vi "Motors Interface.vi"() -> ()   [LabVIEW 2011]
uses:
  Controls/Drive Status.ctl
  <vilib>/LabVIEW Targets/FPGA/cRIO/cRIO-9505/controls.llb/_nicrio_cRIO-9505_DriveStatus.ctl
  <vilib>/Platform/TimedLoop/XDataNode/timing_clust.ctl
  <vilib>/Platform/TimedLoop/XDataNode/nitl_modes.ctl
  <vilib>/Platform/TimedLoop/XDataNode/wakeup.ctl
  Controls/Motor Names.ctl
  Controls/Motor Module.ctl
  Controls/Encoder Module.ctl
  <vilib>/Platform/TimedLoop/XDataNode/XDataNode.xnode
  <vilib>/Platform/TimedLoop/XDataNode/XDNodeRunTimeDep.lvlib
panel:
  in  "tikcs before":i16=10
  out "Current Index 3":i16
  out "Current Index 2":i16
  out "Current Index 1":i16
  out "Current Middle 3":i16
  out "Current Middle 2":i16
  out "Current Middle 1":i16
  out "Current Redundant":i16
  out "Current Thumb 3":i16
  out "Current Thumb 2":i16
  out "Current Thumb 1":i16
  out "Motors Status":T1[](array[typedef])=[{"Status"=enum."Enabled", "Vsup Present"=FALSE, "Drive Fault"=FALSE, "Temp Fault"=FALSE}, {"Status"=enum."Enabled", "Vsup Present"=FALSE, "Drive Fault"=FALSE, "Temp Fault"=FALSE}, {"Status"=enum."Enabled", "Vsup Present"=FALSE, "Drive Fault"=FALSE, "Temp Fault"=FALSE}, {"Status"=enum."Enabled", "Vsup Present"=FALSE, "Drive Fault"=FALSE, "Temp Fault"=FALSE}, {"Status"=enum."Enabled", "Vsup Present"=FALSE, "Drive Fault"=FALSE, "Temp Fault"=FALSE}, {"Status"=enum."Enabled", "Vsup Present"=FALSE, "Drive Fault"=FALSE, "Temp Fault"=FALSE}, {"Status"=enum."Enabled", "Vsup Present"=FALSE, "Drive Fault"=FALSE, "Temp Fault"=FALSE}, {"Status"=enum."Enabled", "Vsup Present"=FALSE, "Drive Fault"=FALSE, "Temp Fault"=FALSE}, {"Status"=enum."Enabled", "Vsup Present"=FALSE, "Drive Fault"=FALSE, "Temp Fault"=FALSE}, {"Status"=enum."Enabled", "Vsup Present"=FALSE, "Drive Fault"=FALSE, "Temp Fault"=FALSE}]
  out "Position Middle 3":i32
  in  "Current Limit Middle 3":i16 caption="Setpoint"
  in  "Current Setpoint Middle 3":i16
  out "Position Middle 2":i32
  in  "Current Limit Middle 2":i16 caption="Setpoint"
  in  "Current Setpoint Middle 2":i16
  out "Position Middle 1":i32
  in  "Current Limit Middle 1":i16 caption="Setpoint"
  in  "Current Setpoint Middle 1":i16
  out "Position Redundant":i32
  in  "Current Limit Redundant":i16 caption="Setpoint"
  in  "Current Setpoint Redundant":i16
  out "Position Thumb 3":i32
  in  "Current Limit Thumb 3":i16 caption="Setpoint"
  in  "Current Setpoint Thumb 3":i16
  out "Position Thumb 2":i32
  in  "Current Limit Thumb 2":i16 caption="Setpoint"
  in  "Current Setpoint Thumb 2":i16
  out "Position Thumb 1":i32
  in  "Current Limit Thumb 1":i16 caption="Setpoint"
  in  "Current Setpoint Thumb 1":i16
  out "Position Index 3":i32
  in  "Current Limit Index 3":i16 caption="Setpoint"
  in  "Current Setpoint Index 3":i16
  out "Position Index 2":i32
  in  "Current Limit Index 2":i16 caption="Setpoint"
  in  "Current Setpoint Index 2":i16
  out "Position Index 1":i32
  in  "Current Limit Index 1":i16 caption="Setpoint"
  in  "Rate (usec)":u32=50
  in  "Motors Gains":T3={"Proportional Gain"=20, "Integral Gain"=10, "Derivative Gain"=0}
  in  "Current Setpoint Index 1":i16
  out "All Enabled":bool
  in  "Disable\nMotors":bool
  in  "Enable\nMotors":bool
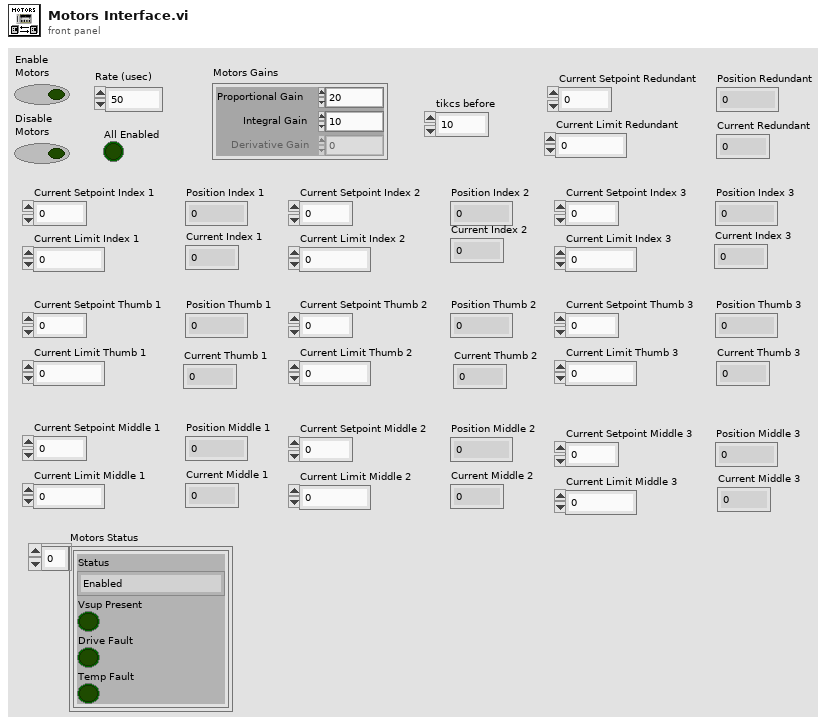
[diagram p1: front panel]
types:
  T1 = typedef "Drive Status.ctl" = cluster{"Status":T2, "Vsup Present":bool, "Drive Fault":bool, "Temp Fault":bool}
  T2 = typedef "_nicrio_cRIO-9505_DriveStatus.ctl" = enum8{"Enabled", "Disabled", "Disabled by Drive Fault", "Disabled by Temp. Fault", "Disabled by E-Stop", "Unknown"}
  T3 = cluster{"Proportional Gain":i16, "Integral Gain":i16, "Derivative Gain":i16}
  T4 = typedef "Motor Names.ctl" = enum16{"Thumb1", "Thumb2", "Thumb3", "Middle1", "Middle2", "Middle3", "Redundant", "Index1", "Index2", "Index3"}
  T5 = typedef "XDNodeRunTimeDep.lvlib/timing_clust.ctl" = cluster{"Expected End [f-1]":u64, "Actual End [f-1]":u64, "Finished Late? [f-1]":bool, "Expected End [i-1]":u64, "Actual End [i-1]":u64, "Finished Late? [i-1]":bool, "Expected Start [i]":u64, "Actual Start [i]":u64, "Expected Start [f]":u64, "Actual Start [f]":u64, "Source Name":string, "Structure Name":string, "Period":i64, "Deadline":i64, "Offset":i64, "Start":i64, "Priority":i32, "Timeout":i32, "Mode":T6, "Wakeup Reason":T7, "Error":errorcluster, "Source Type":string, "Secondary Source Type":string, "Global End Time":u64, "Global Start Time":u64, "Frame Duration":u64, "Iteration Duration":u64, "Assigned CPU":i32, "I/O Scan Engine Mode":u32}
  T6 = typedef "XDNodeRunTimeDep.lvlib/nitl_modes.ctl" = enum32{"No Change", "Process missed periods, maintain original phase", "Discard missed periods, maintain original phase", "Process missed periods, ignore original phase", "Discard missed periods, ignore original phase"}
  T7 = typedef "XDNodeRunTimeDep.lvlib/wakeup.ctl" = enum32{"Normal", "Aborted", "Asynchronous wakeup", "Timing source error", "Timed loop error", "Timeout"}
  T8 = typedef "Encoder Module.ctl" = cluster{"Encoder Phase A":refnum<k21>, "Encoder Phase B":refnum<k21>, "Encoder Index":refnum<k21>}
  T9 = typedef "Motor Module.ctl" = cluster{"Motor":refnum<k21>, "Drive Direction":refnum<k21>}
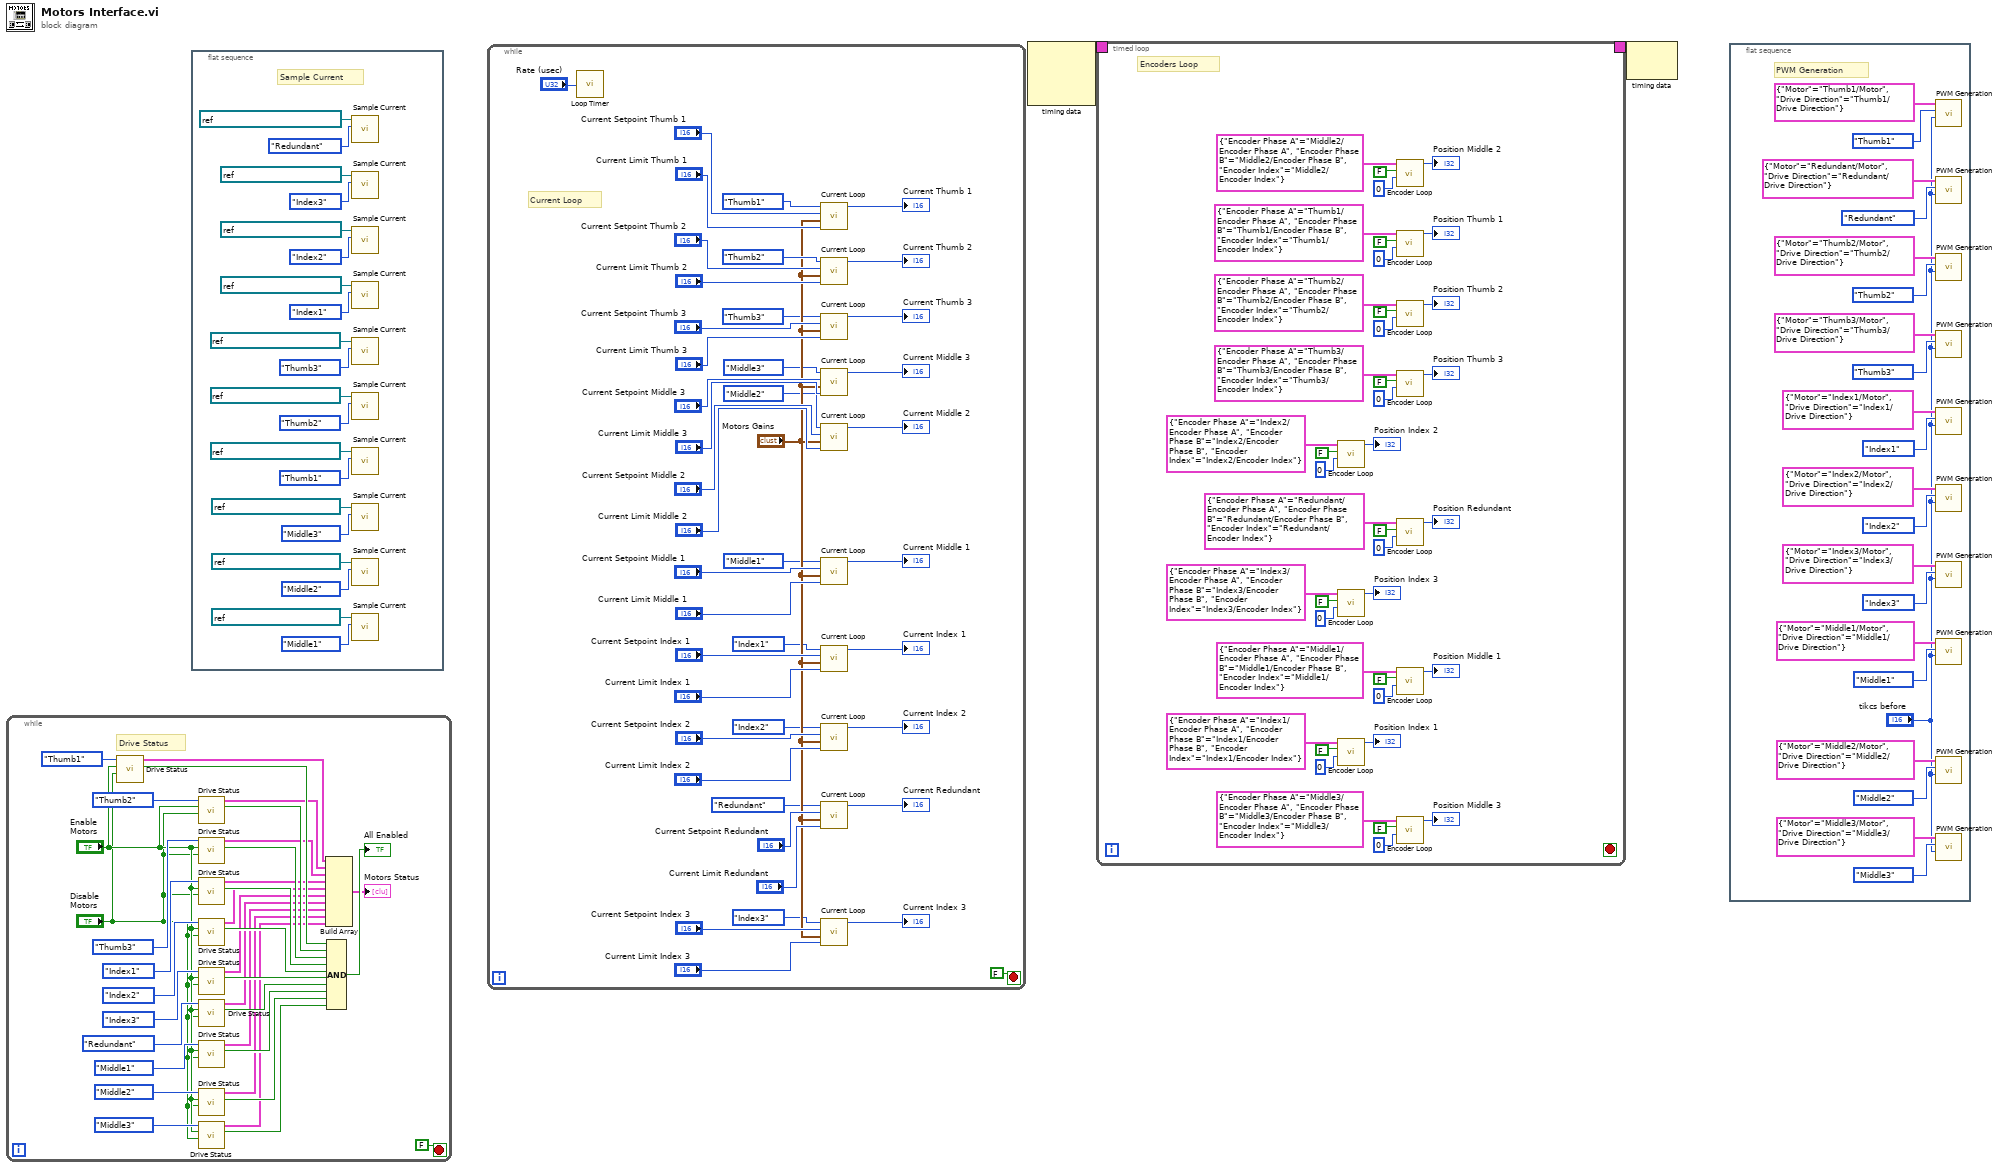
[diagram p0: block diagram]
diagram:
  n1 = while {
    stop <- FALSE stop-if-true
    # "Drive Status"
    n2 = call "Drive Status.vi"("Disable\nDrive"="Disable\nMotors", "Enable\nDrive"="Enable\nMotors", "Motor"=Motor_Names."Thumb1") -> ("Enabled?"=w24:bool, "Drive Status"=w14:T1)  [unwired: 7 in]
    n3 = call "Drive Status.vi"("Disable\nDrive"="Disable\nMotors", "Enable\nDrive"="Enable\nMotors", "Motor"=Motor_Names."Thumb2") -> ("Enabled?"=w23:bool, "Drive Status"=w13:T1)  [unwired: 7 in]
    n4 = call "Drive Status.vi"("Disable\nDrive"="Disable\nMotors", "Enable\nDrive"="Enable\nMotors", "Motor"=Motor_Names."Thumb3") -> ("Enabled?"=w22:bool, "Drive Status"=w12:T1)  [unwired: 7 in]
    n5 = call "Drive Status.vi"("Disable\nDrive"="Disable\nMotors", "Enable\nDrive"="Enable\nMotors", "Motor"=Motor_Names."Index1") -> ("Enabled?"=w21:bool, "Drive Status"=w11:T1)  [unwired: 7 in]
    n6 = call "Drive Status.vi"("Disable\nDrive"="Disable\nMotors", "Enable\nDrive"="Enable\nMotors", "Motor"=Motor_Names."Index2") -> ("Enabled?"=w20:bool, "Drive Status"=w10:T1)  [unwired: 7 in]
    n7 = call "Drive Status.vi"("Disable\nDrive"="Disable\nMotors", "Enable\nDrive"="Enable\nMotors", "Motor"=Motor_Names."Index3") -> ("Enabled?"=w19:bool, "Drive Status"=w9:T1)  [unwired: 7 in]
    n8 = call "Drive Status.vi"("Disable\nDrive"="Disable\nMotors", "Enable\nDrive"="Enable\nMotors", "Motor"=Motor_Names."Redundant") -> ("Enabled?"=w18:bool, "Drive Status"=w8:T1)  [unwired: 7 in]
    n9 = call "Drive Status.vi"("Disable\nDrive"="Disable\nMotors", "Enable\nDrive"="Enable\nMotors", "Motor"=Motor_Names."Middle1") -> ("Enabled?"=w17:bool, "Drive Status"=w7:T1)  [unwired: 7 in]
    n10 = call "Drive Status.vi"("Disable\nDrive"="Disable\nMotors", "Enable\nDrive"="Enable\nMotors", "Motor"=Motor_Names."Middle2") -> ("Enabled?"=w16:bool, "Drive Status"=w6:T1)  [unwired: 7 in]
    n11 = call "Drive Status.vi"("Disable\nDrive"="Disable\nMotors", "Enable\nDrive"="Enable\nMotors", "Motor"=Motor_Names."Middle3") -> ("Enabled?"=w15:bool, "Drive Status"=w5:T1)  [unwired: 7 in]
    n12 = Build Array(w14, w13, w12, w11, w10, w9, w8, w7, w6, w5) -> (→"Motors Status":T1[])
    n13 = Compound Arithmetic op=AND(w24, w23, w22, w21, w20, w19, w18, w17, w16, w15) -> (→"All Enabled":bool)
  }
  n14 = flat-sequence {
    frame #0 {
      # "Sample Current"
      n15 = call "Sample Current.vi"("Motor Index"=Motor_Names."Redundant" ("Motor Names"), "Current Sense I/O"=refnum<k21> "Redundant/Current Sense") -> ()  [unwired: 10 in]
      n16 = call "Sample Current.vi"("Motor Index"=Motor_Names."Index3" ("Motor Names"), "Current Sense I/O"=refnum<k21> "Index3/Current Sense") -> ()  [unwired: 10 in]
      n17 = call "Sample Current.vi"("Motor Index"=Motor_Names."Index2" ("Motor Names"), "Current Sense I/O"=refnum<k21> "Index2/Current Sense") -> ()  [unwired: 10 in]
      n18 = call "Sample Current.vi"("Motor Index"=Motor_Names."Index1" ("Motor Names"), "Current Sense I/O"=refnum<k21> "Index1/Current Sense") -> ()  [unwired: 10 in]
      n19 = call "Sample Current.vi"("Motor Index"=Motor_Names."Thumb3" ("Motor Names"), "Current Sense I/O"=refnum<k21> "Thumb3/Current Sense") -> ()  [unwired: 10 in]
      n20 = call "Sample Current.vi"("Motor Index"=Motor_Names."Thumb2" ("Motor Names"), "Current Sense I/O"=refnum<k21> "Thumb2/Current Sense") -> ()  [unwired: 10 in]
      n21 = call "Sample Current.vi"("Motor Index"=Motor_Names."Thumb1" ("Motor Names"), "Current Sense I/O"=refnum<k21> "Thumb1/Current Sense") -> ()  [unwired: 10 in]
      n22 = call "Sample Current.vi"("Motor Index"=Motor_Names."Middle3" ("Motor Names"), "Current Sense I/O"=refnum<k21> "Middle3/Current Sense") -> ()  [unwired: 10 in]
      n23 = call "Sample Current.vi"("Motor Index"=Motor_Names."Middle2" ("Motor Names"), "Current Sense I/O"=refnum<k21> "Middle2/Current Sense") -> ()  [unwired: 10 in]
      n24 = call "Sample Current.vi"("Motor Index"=Motor_Names."Middle1" ("Motor Names"), "Current Sense I/O"=refnum<k21> "Middle1/Current Sense") -> ()  [unwired: 10 in]
    }
  }
  n25 = while {
    stop <- FALSE stop-if-true
    # "Current Loop"
    n26 = call "Loop Timer"("Count(uSec)"="Rate (usec)") -> ()  [unwired: 1 out]
    n27 = call "Current Loop.vi"("Current Limit"="Current Limit Thumb 1", "Gains"="Motors Gains", "Current Setpoint"="Current Setpoint Thumb 1", "Motor Index"=Motor_Names."Thumb1" ("Motor Names")) -> ("Current"=→"Current Thumb 1":i16)  [unwired: 7 in]
    n28 = call "Current Loop.vi"("Current Limit"="Current Limit Thumb 2", "Gains"="Motors Gains", "Current Setpoint"="Current Setpoint Thumb 2", "Motor Index"=Motor_Names."Thumb2" ("Motor Names")) -> ("Current"=→"Current Thumb 2":i16)  [unwired: 7 in]
    n29 = call "Current Loop.vi"("Current Limit"="Current Limit Thumb 3", "Gains"="Motors Gains", "Current Setpoint"="Current Setpoint Thumb 3", "Motor Index"=Motor_Names."Thumb3" ("Motor Names")) -> ("Current"=→"Current Thumb 3":i16)  [unwired: 7 in]
    n30 = call "Current Loop.vi"("Current Limit"="Current Limit Middle 3", "Gains"="Motors Gains", "Current Setpoint"="Current Setpoint Middle 3", "Motor Index"=Motor_Names."Middle3" ("Motor Names")) -> ("Current"=→"Current Middle 3":i16)  [unwired: 7 in]
    n31 = call "Current Loop.vi"("Current Limit"="Current Limit Middle 2", "Gains"="Motors Gains", "Current Setpoint"="Current Setpoint Middle 2", "Motor Index"=Motor_Names."Middle2" ("Motor Names")) -> ("Current"=→"Current Middle 2":i16)  [unwired: 7 in]
    n32 = call "Current Loop.vi"("Current Limit"="Current Limit Middle 1", "Gains"="Motors Gains", "Current Setpoint"="Current Setpoint Middle 1", "Motor Index"=Motor_Names."Middle1" ("Motor Names")) -> ("Current"=→"Current Middle 1":i16)  [unwired: 7 in]
    n33 = call "Current Loop.vi"("Current Limit"="Current Limit Index 1", "Gains"="Motors Gains", "Current Setpoint"="Current Setpoint Index 1", "Motor Index"=Motor_Names."Index1" ("Motor Names")) -> ("Current"=→"Current Index 1":i16)  [unwired: 7 in]
    n34 = call "Current Loop.vi"("Current Limit"="Current Limit Index 2", "Gains"="Motors Gains", "Current Setpoint"="Current Setpoint Index 2", "Motor Index"=Motor_Names."Index2" ("Motor Names")) -> ("Current"=→"Current Index 2":i16)  [unwired: 7 in]
    n35 = call "Current Loop.vi"("Current Limit"="Current Limit Redundant", "Gains"="Motors Gains", "Current Setpoint"="Current Setpoint Redundant", "Motor Index"=Motor_Names."Redundant" ("Motor Names")) -> ("Current"=→"Current Redundant":i16)  [unwired: 7 in]
    n36 = call "Current Loop.vi"("Current Limit"="Current Limit Index 3", "Gains"="Motors Gains", "Current Setpoint"="Current Setpoint Index 3", "Motor Index"=Motor_Names."Index3" ("Motor Names")) -> ("Current"=→"Current Index 3":i16)  [unwired: 7 in]
  }
  n37 = node-c288() -> (w2:T5)  [unwired: 2 in, 1 out]
  n38 = timed-loop {
    timing: w2 -> [_]
    timing-out: [_] -> w1
    stop <- _ stop-if-true
    # "Encoders Loop"
    n39 = call "Encoder Loop.vi"("Reset Position Value"=0, "Reset Position"=FALSE, "Motor Module"=T8 {"Encoder Phase A"="Index2/Encoder Phase A", "Encoder Phase B"="Index2/Encoder Phase B", "Encoder Index"="Index2/Encoder Index"} ("Encoder Module")) -> ("Encoder Position"=→"Position Index 2":i32)  [unwired: 5 in, 3 out]
    n40 = call "Encoder Loop.vi"("Reset Position Value"=0, "Reset Position"=FALSE, "Motor Module"=T8 {"Encoder Phase A"="Index3/Encoder Phase A", "Encoder Phase B"="Index3/Encoder Phase B", "Encoder Index"="Index3/Encoder Index"} ("Encoder Module")) -> ("Encoder Position"=→"Position Index 3":i32)  [unwired: 5 in, 3 out]
    n41 = call "Encoder Loop.vi"("Reset Position Value"=0, "Reset Position"=FALSE, "Motor Module"=T8 {"Encoder Phase A"="Index1/Encoder Phase A", "Encoder Phase B"="Index1/Encoder Phase B", "Encoder Index"="Index1/Encoder Index"} ("Encoder Module")) -> ("Encoder Position"=→"Position Index 1":i32)  [unwired: 5 in, 3 out]
    n42 = call "Encoder Loop.vi"("Reset Position Value"=0, "Reset Position"=FALSE, "Motor Module"=T8 {"Encoder Phase A"="Middle2/Encoder Phase A", "Encoder Phase B"="Middle2/Encoder Phase B", "Encoder Index"="Middle2/Encoder Index"} ("Encoder Module")) -> ("Encoder Position"=→"Position Middle 2":i32)  [unwired: 5 in, 3 out]
    n43 = call "Encoder Loop.vi"("Reset Position Value"=0, "Reset Position"=FALSE, "Motor Module"=T8 {"Encoder Phase A"="Thumb1/Encoder Phase A", "Encoder Phase B"="Thumb1/Encoder Phase B", "Encoder Index"="Thumb1/Encoder Index"} ("Encoder Module")) -> ("Encoder Position"=→"Position Thumb 1":i32)  [unwired: 5 in, 3 out]
    n44 = call "Encoder Loop.vi"("Reset Position Value"=0, "Reset Position"=FALSE, "Motor Module"=T8 {"Encoder Phase A"="Thumb2/Encoder Phase A", "Encoder Phase B"="Thumb2/Encoder Phase B", "Encoder Index"="Thumb2/Encoder Index"} ("Encoder Module")) -> ("Encoder Position"=→"Position Thumb 2":i32)  [unwired: 5 in, 3 out]
    n45 = call "Encoder Loop.vi"("Reset Position Value"=0, "Reset Position"=FALSE, "Motor Module"=T8 {"Encoder Phase A"="Thumb3/Encoder Phase A", "Encoder Phase B"="Thumb3/Encoder Phase B", "Encoder Index"="Thumb3/Encoder Index"} ("Encoder Module")) -> ("Encoder Position"=→"Position Thumb 3":i32)  [unwired: 5 in, 3 out]
    n46 = call "Encoder Loop.vi"("Reset Position Value"=0, "Reset Position"=FALSE, "Motor Module"=T8 {"Encoder Phase A"="Redundant/Encoder Phase A", "Encoder Phase B"="Redundant/Encoder Phase B", "Encoder Index"="Redundant/Encoder Index"} ("Encoder Module")) -> ("Encoder Position"=→"Position Redundant":i32)  [unwired: 5 in, 3 out]
    n47 = call "Encoder Loop.vi"("Reset Position Value"=0, "Reset Position"=FALSE, "Motor Module"=T8 {"Encoder Phase A"="Middle1/Encoder Phase A", "Encoder Phase B"="Middle1/Encoder Phase B", "Encoder Index"="Middle1/Encoder Index"} ("Encoder Module")) -> ("Encoder Position"=→"Position Middle 1":i32)  [unwired: 5 in, 3 out]
    n48 = call "Encoder Loop.vi"("Reset Position Value"=0, "Reset Position"=FALSE, "Motor Module"=T8 {"Encoder Phase A"="Middle3/Encoder Phase A", "Encoder Phase B"="Middle3/Encoder Phase B", "Encoder Index"="Middle3/Encoder Index"} ("Encoder Module")) -> ("Encoder Position"=→"Position Middle 3":i32)  [unwired: 5 in, 3 out]
  }
  n49 = node-c288(w1) -> ()  [unwired: 1 out]
  n50 = flat-sequence {
    frame #0 {
      # "PWM Generation"
      n51 = call "PWM Generation.vi"("tikcs before"="tikcs before", "Motor Index"=Motor_Names."Thumb1" ("Motor Names"), "Motor Module"=T9 {"Motor"="Thumb1/Motor", "Drive Direction"="Thumb1/Drive Direction"}) -> ()  [unwired: 9 in]
      n52 = call "PWM Generation.vi"("tikcs before"="tikcs before", "Motor Index"=Motor_Names."Redundant" ("Motor Names"), "Motor Module"=T9 {"Motor"="Redundant/Motor", "Drive Direction"="Redundant/Drive Direction"}) -> ()  [unwired: 9 in]
      n53 = call "PWM Generation.vi"("tikcs before"="tikcs before", "Motor Index"=Motor_Names."Thumb2" ("Motor Names"), "Motor Module"=T9 {"Motor"="Thumb2/Motor", "Drive Direction"="Thumb2/Drive Direction"}) -> ()  [unwired: 9 in]
      n54 = call "PWM Generation.vi"("tikcs before"="tikcs before", "Motor Index"=Motor_Names."Thumb3" ("Motor Names"), "Motor Module"=T9 {"Motor"="Thumb3/Motor", "Drive Direction"="Thumb3/Drive Direction"}) -> ()  [unwired: 9 in]
      n55 = call "PWM Generation.vi"("tikcs before"="tikcs before", "Motor Index"=Motor_Names."Index1" ("Motor Names"), "Motor Module"=T9 {"Motor"="Index1/Motor", "Drive Direction"="Index1/Drive Direction"}) -> ()  [unwired: 9 in]
      n56 = call "PWM Generation.vi"("tikcs before"="tikcs before", "Motor Index"=Motor_Names."Index2" ("Motor Names"), "Motor Module"=T9 {"Motor"="Index2/Motor", "Drive Direction"="Index2/Drive Direction"}) -> ()  [unwired: 9 in]
      n57 = call "PWM Generation.vi"("tikcs before"="tikcs before", "Motor Index"=Motor_Names."Index3" ("Motor Names"), "Motor Module"=T9 {"Motor"="Index3/Motor", "Drive Direction"="Index3/Drive Direction"}) -> ()  [unwired: 9 in]
      n58 = call "PWM Generation.vi"("tikcs before"="tikcs before", "Motor Index"=Motor_Names."Middle1" ("Motor Names"), "Motor Module"=T9 {"Motor"="Middle1/Motor", "Drive Direction"="Middle1/Drive Direction"}) -> ()  [unwired: 9 in]
      n59 = call "PWM Generation.vi"("tikcs before"="tikcs before", "Motor Index"=Motor_Names."Middle2" ("Motor Names"), "Motor Module"=T9 {"Motor"="Middle2/Motor", "Drive Direction"="Middle2/Drive Direction"}) -> ()  [unwired: 9 in]
      n60 = call "PWM Generation.vi"("tikcs before"="tikcs before", "Motor Index"=Motor_Names."Middle3" ("Motor Names"), "Motor Module"=T9 {"Motor"="Middle3/Motor", "Drive Direction"="Middle3/Drive Direction"}) -> ()  [unwired: 9 in]
    }
  }
